vi "Recieve Request.vi"(8 "error in (no error)":errorcluster, 10 "Device Connector MSG In":refnum<class "Device Connector MSG.lvclass">, 11 "Device Connector in":refnum<class "Device Connector.lvclass">) -> (0 "error out":errorcluster, 3 "Device Connector out":refnum<class "Device Connector.lvclass">)   [LabVIEW 2024, in "Device Connector.lvclass"]
uses:
  Device Connector.lvclass
  Device Connector MSG/Device Connector MSG.lvclass
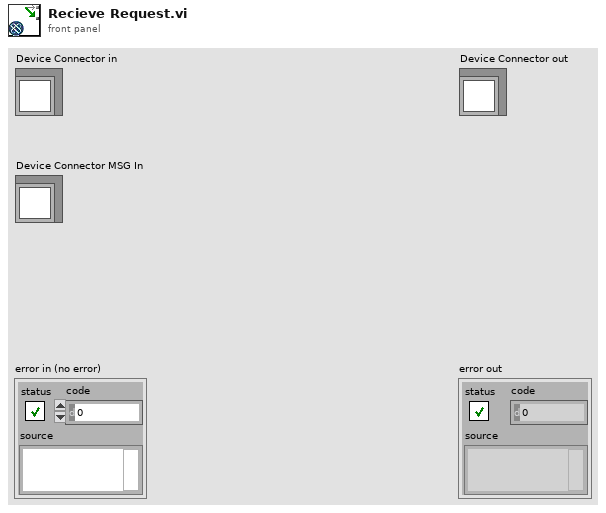
[diagram p1: front panel]
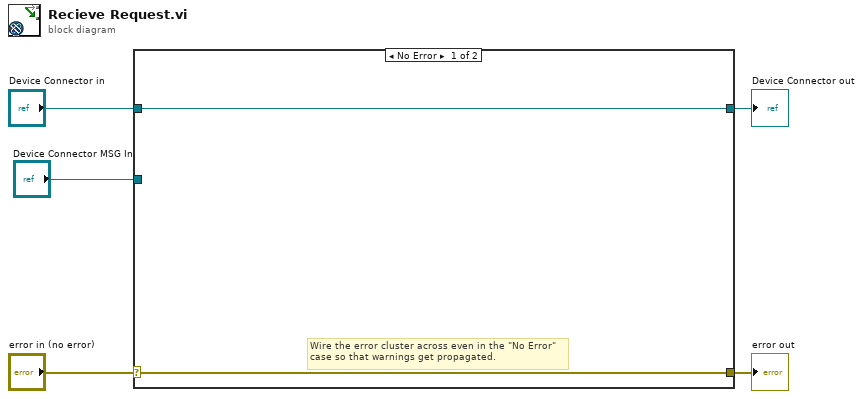
[diagram p0: block diagram]
diagram:
  n1 = case shown="No Error" "error in (no error)" {
    selector: "error in (no error)" -> [w6 w9]
    tunnel: [w6 w9] -> w4
    tunnel: [w7 w8] -> w2
    tunnel: "Device Connector in" -> [w7 w8]
    tunnel: "Device Connector MSG In" -> [_ _]
    frame No Error {
      # "Wire the error cluster across even in the \"No Error\"\ncase so that warnings get propagated."
    }
    frame Error {
    }
  }
  "error out" <- w4
  "Device Connector out" <- w2
